vi "uTTA_DeleteFile.vi"(4 "error in":errorcluster, 6 "Directory Name":string="\\", 7 "VISA Refnum in":refnum<visa-resource-name>) -> (0 "error out":errorcluster, 2 "Received":string, 3 "VISA Refnum out":refnum<visa-resource-name>)   [LabVIEW 2021]
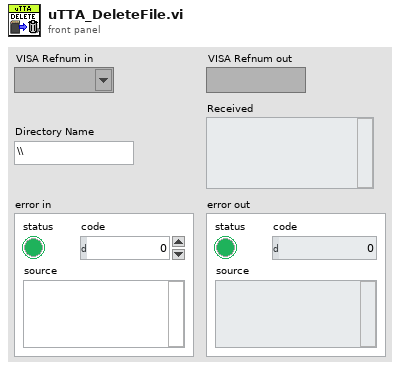
[diagram p1: front panel]
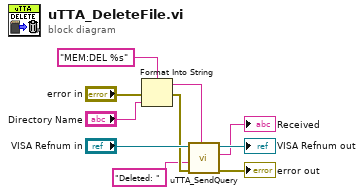
[diagram p0: block diagram]
diagram:
  n1 = Format Into String(format string="MEM:DEL %s", error in="error in", "Directory Name") -> (resulting string=w7:string, error out=w6:errorcluster)  [unwired: 1 in]
  n2 = call "uTTA_SendQuery.vi"("Send String"=w7, "error in (no error)"=w6, "Response Qualifier(\"\")"="Deleted: " ("Response Qualifier(\"\")"), "VISA Refnum in"="VISA Refnum in") -> ("error out"=→"error out":errorcluster, "Received"=→"Received":string, "VISA Refnum out"=→"VISA Refnum out":refnum<visa-resource-name>)  [unwired: 5 in]
